vi "SOLA Control.vi"() -> ()   [LabVIEW 2018]
uses:
  <vilib>/LUMENCOR/Lumencor DLL 4.1.x (64bit)/LumencorDLL64.lvlib
panel:
  in  "Intensity [%]":u16(slide) scale=0.0..100.0 scale format="%.1f"
  in  "Combo Box":string(combo)="OFF"
  in  "stop":bool
  out "error out 2":errorcluster
  out "LETypeStr out":string
  in  "ComPort":i32=5
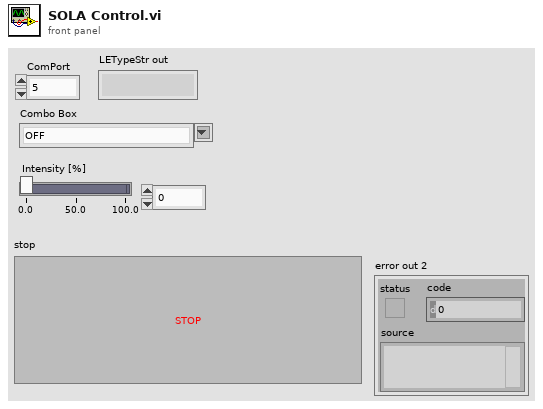
[diagram p1: front panel]
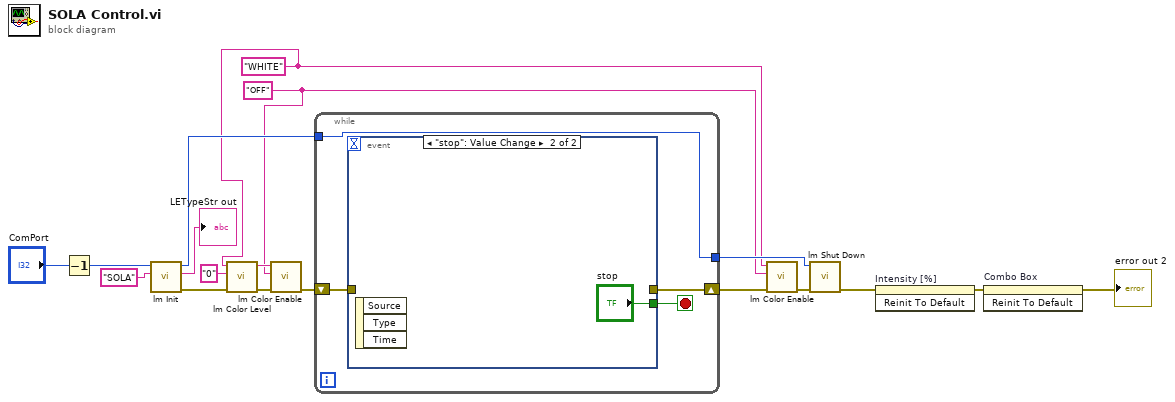
[diagram p0: block diagram]
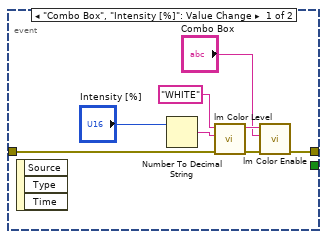
[diagram p2: hidden frame]
diagram:
  w6 = "OFF" ("str_State")
  w5 = "WHITE"
  n1 = Decrement(x="ComPort") -> (x-1=w17:i32)
  n2 = call <vilib>:"lm Init.vi"("LETypeStr"="SOLA", "ComPort"=w17) -> ("error out"=w8:errorcluster, "LETypeStr out"=→"LETypeStr out":string, "function return"=w11:u32)  [unwired: 7 in]
  n3 = call <vilib>:"lm Color Level.vi"("error in (no error)"=w8, "str_Level"="0", "str_Color"=w5) -> ("error out"=w10:errorcluster, "str_Color out"=w9:string)  [unwired: 6 in, 1 out]
  n4 = call <vilib>:"lm Color Enable.vi"("error in (no error)"=w10, "str_State"=w6, "str_Color"=w9) -> ("error out"=w7:errorcluster)  [unwired: 6 in, 2 out]
  n5 = while {
    tunnel: [w22] -> w18
    tunnel: w11 -> [w22]
    shift-right: [w20] -> w15
    shift-left: w7 -> [w21]
    stop <- w19 stop-if-true
    n6 = event shown="[1] \"stop\": Value Change" {
      selector: _ -> [_ _]
      dyn-events: _ -> [_ _]
      timeout: _ -> [_ _]
      tunnel: w21 -> [w26 _]
      tunnel: [w24 _] -> w20
      tunnel: [_ "stop"] -> w19
      event "Combo Box", "Intensity [%]": Value Change {
        n7 = event-data() -> ()  [unwired: 1 in, 3 out]
        n8 = Number To Decimal String(number="Intensity [%]") -> (decimal integer string=w30:string)  [unwired: 1 in]
        n9 = call <vilib>:"lm Color Level.vi"("error in (no error)"=w26, "str_Level"=w30, "str_Color"="WHITE") -> ("error out"=w27:errorcluster, "str_Color out"=w28:string)  [unwired: 6 in, 1 out]
        n10 = call <vilib>:"lm Color Enable.vi"("error in (no error)"=w27, "str_State"="Combo Box", "str_Color"=w28) -> ("error out"=w24:errorcluster)  [unwired: 6 in, 2 out]
      }
      event "stop": Value Change {
        n11 = event-data() -> ()  [unwired: 1 in, 3 out]
      }
    }
  }
  n12 = call <vilib>:"lm Color Enable.vi"("error in (no error)"=w15, "str_State"=w6, "str_Color"=w5) -> ("error out"=w14:errorcluster)  [unwired: 6 in, 2 out]
  n13 = call <vilib>:"lm Shut Down.vi"("error in (no error)"=w14, "hSerial"=w18) -> ("error out"=w3:errorcluster)  [unwired: 8 in, 1 out]
  n14 = invoke on="Intensity [%]" class="Slide (strict)" method="Reinit To Default"(error in=w3) -> (error out=w2:errorcluster)  [unwired: 2 in, 2 out]
  n15 = invoke on="Combo Box" class="CmbBox" method="Reinit To Default"(error in=w2) -> (error out=→"error out 2":errorcluster)  [unwired: 2 in, 2 out]
